vi "Build v2.vi"(7 "buffer conversion descriptor":T1 {"conversions"."converted descriptor"."buffer offset" format="%d bytes"; "conversions"."unconverted descriptor"."buffer offset" format="%d bytes"}, 8 "error in (no error)":errorcluster, 9 "dst Buffer":refnum<class "Buffer.lvclass">, 10 "src Buffer":refnum<class "Buffer.lvclass">, 11 "Buffer Converter in":refnum<class "Buffer Converter.lvclass">) -> (0 "error out":errorcluster, 3 "Buffer Converter out":refnum<class "Buffer Converter.lvclass">)   [LabVIEW 2017, in "DSF Core.lvlib" / "Buffer Converter.lvclass"]
uses:
  Buffer Converter.lvclass
  Buffer/Buffer.lvclass
  Buffer/Read Buffer String.vi
  Buffer/Write Buffer String.vi
  DSF Configuration API/Public/Controls/DSF Data Type.ctl
  DSF Core.lvlib
  Channel Descriptor.ctl
  Conversion.ctl
  Buffer Conversion Descriptor.ctl
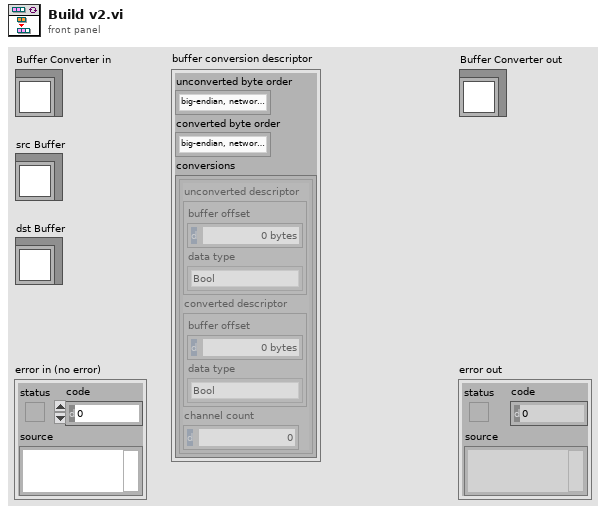
[diagram p1: front panel]
types:
  T1 = typedef "DSF Core.lvlib/Buffer Converter.lvclass/Buffer Conversion Descriptor.ctl" = cluster{"unconverted byte order":enum16{"big-endian, network order", "native, host order", "little-endian"}, "converted byte order":enum16{"big-endian, network order", "native, host order", "little-endian"}, "conversions":T2[]}
  T2 = typedef "DSF Core.lvlib/Buffer Converter.lvclass/Conversion.ctl" = cluster{"unconverted descriptor":T3, "converted descriptor":T3, "channel count":u64}
  T3 = typedef "DSF Core.lvlib/Buffer Converter.lvclass/Channel Descriptor.ctl" = cluster{"buffer offset":u64, "data type":T4}
  T4 = typedef "DSF Core.lvlib/DSF Data Type.ctl" = enum8{"Bool", "SGL", "DBL", "I8", "I16", "I32", "I64", "U8", "U16", "U32", "U64"}
  T5 = enum16{"big-endian, network order", "native, host order", "little-endian"}
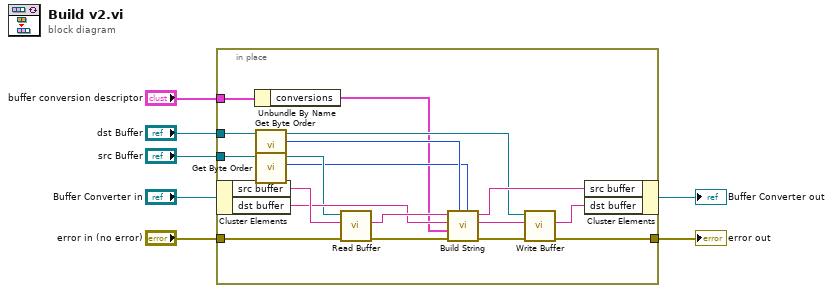
[diagram p0: block diagram]
diagram:
  n1 = in-place {
    in-place-border: "src Buffer" -> [w14]
    in-place-border: "dst Buffer" -> [w12]
    in-place-border: [w24] -> w5
    in-place-border: "error in (no error)" -> [w22]
    in-place-border: "buffer conversion descriptor" -> [w15]
    n2 = in-place-cluster #1("Buffer Converter in") -> ("src buffer"=w21:string, "dst buffer"=w19:string)
    n3 = Unbundle By Name(w15) -> ("conversions"=w8:T2[])
    n4 = call "Get Byte Order.vi"("Buffer in"=w12) -> ("byte order"=w10:T5, "Buffer out"=w11:refnum<class "Buffer.lvclass">)  [unwired: 9 in]
    n5 = call "Get Byte Order.vi"("Buffer in"=w14) -> ("byte order"=w9:T5, "Buffer out"=w13:refnum<class "Buffer.lvclass">)  [unwired: 9 in]
    n6 = call-poly "Read Buffer.vi"("error in (no error)"=w22, "buffer in"=w21, "Buffer in"=w13) -> ("error out"=w23:errorcluster, "buffer out"=w20:string)  [unwired: 5 in, 2 out]
    n7 = call "Build String.vi"("src byte order"=w9, "dst byte order"=w10, "error in (no error)"=w23, "conversions"=w8, "dst buffer in"=w19, "src buffer in"=w20) -> ("error out"=w25:errorcluster, "dst buffer out"=w17:string, "src buffer out"=w18:string)  [unwired: 3 in]
    n8 = call-poly "Write Buffer.vi"("error in (no error)"=w25, "buffer in"=w17, "Buffer in"=w11) -> ("error out"=w24:errorcluster, "buffer out"=w16:string)  [unwired: 5 in, 2 out]
    n9 = in-place-cluster #1("src buffer"=w18, "dst buffer"=w16) -> (→"Buffer Converter out":refnum<class "Buffer Converter.lvclass">)
  }
  "error out" <- w5
